vi "saveImage.vi"(8 "error in (no error)":errorcluster, 10 "URI":string, 11 "Camera.Simulated":refnum<class "Camera.Simulated.lvclass">) -> (0 "error out":errorcluster, 3 "Camera.Simulated out":refnum<class "Camera.Simulated.lvclass">)   [LabVIEW 2015]
doc: "---------------------------------------------------------------\nJKI State Machine Objects™\nhttp://jki.net/state-machine-objects/\nCopyright (C) 2005-2015, JKI <info@jki.net>\nALL RIGHTS RESERVEDJKI State Machine Objects (SMO) 1.0.0.5\nJKI - JKI\nCopyright (c) 2016, JKI"
uses:
  Camera.Simulated.lvclass
  <userlib>/_OpenG.lib/file/file.llb/Strip Path Extension - Path__ogtk.vi
panel:
  # "For instructions on how to use the JKI State Machine Objects, examples and video tutorials, visit:\nhttp://jki.net/state-machine-objects/\n\nJKI State Machine Objects™\nhttp://jki.net/state-machine-objects/\nCopyright (C) 2005-2015, JKI <info@jki.net>\nALL RIGHTS RESERVED"
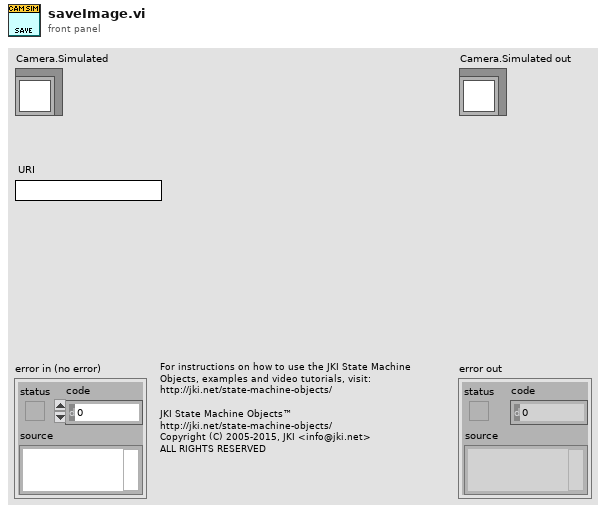
[diagram p1: front panel]
types:
  T1 = typedef "imagedata.ctl" = cluster{"image type":i32, "image depth":i32, "image":u8[], "mask":u8[], "colors":u32[], "Rectangle":cluster{"left":i16, "top":i16, "right":i16, "bottom":i16}}
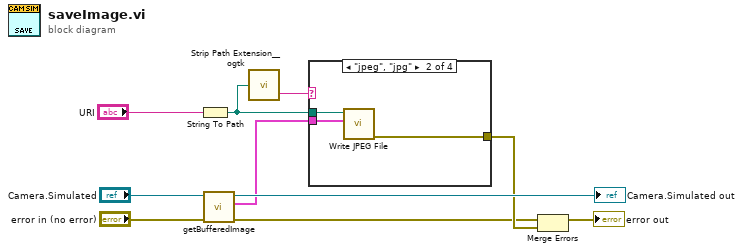
[diagram p0: block diagram]
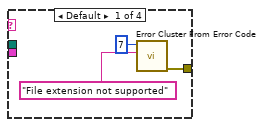
[diagram p2: hidden frame]
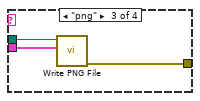
[diagram p3: hidden frame]
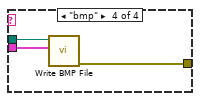
[diagram p4: hidden frame]
diagram:
  n1 = String To Path(string="URI") -> (path=w4:path)
  n2 = call-dynamic "getBufferedImage.vi"("error in (no error)"="error in (no error)", "Camera.Simulated in"="Camera.Simulated") -> ("error out"=w2:errorcluster, "image data"=w5:T1, "Camera.Simulated out"=→"Camera.Simulated out":refnum<class "Camera.Simulated.lvclass">)  [unwired: 7 in]
  n3 = call-poly <userlib>:"Strip Path Extension__ogtk.vi"("path"=w4) -> ("extension"=w6:string)  [unwired: 1 out]
  n4 = case shown="\"jpeg\", \"jpg\"" w6 {
    tunnel: w5 -> [_ w16 w18 w21]
    tunnel: w4 -> [_ w15 w19 w22]
    tunnel: [w13 w14 w17 w20] -> w3
    frame Default {
      n5 = call <vilib>:"Error Cluster From Error Code.vi"("error message (\"\")"="File extension not supported", "error code (0)"=7) -> ("error out"=w13:errorcluster)  [unwired: 7 in]
    }
    frame "jpeg", "jpg" {
      n6 = call <vilib>:"Write JPEG File.vi"("image data"=w16, "path to JPEG file"=w15) -> ("error out"=w14:errorcluster)  [unwired: 8 in, 1 out]
    }
    frame "png" {
      n7 = call <vilib>:"Write PNG File.vi"("image data"=w18, "path to PNG file"=w19) -> ("error out"=w17:errorcluster)  [unwired: 8 in, 1 out]
    }
    frame "bmp" {
      n8 = call <vilib>:"Write BMP File.vi"("image data"=w21, "path to BMP file"=w22) -> ("error out"=w20:errorcluster)  [unwired: 8 in, 1 out]
    }
  }
  n9 = Merge Errors(w2, w3) -> (→"error out":errorcluster)
